vi "Write FXP.vi"(7 "FXP Configuration":T1, 8 "error in":errorcluster, 9 "DBL Value":dbl, 10 "register name":string, 11 "session in":u32) -> (0 "error out":errorcluster, 3 "session out":u32)   [LabVIEW 2018, in "FPGA Register IO.lvlib"]
uses:
  FPGA Register IO.lvlib
  TypeDefs/FXP Configuration.ctl
  <vilib>/fxp/LVFixedPointRepBitsTypeDef.ctl
  <vilib>/fxp/LVFixedPointRepRangeTypeDef.ctl
  Utilities/Find Register Offset.vi
  SubVIs/Check Register Data Store.vi
  Error Handling/Error 6001.vi
  Error Handling/Error 6000.vi
  Error Handling/Error 6002.vi
  Error Handling/Error 6006.vi
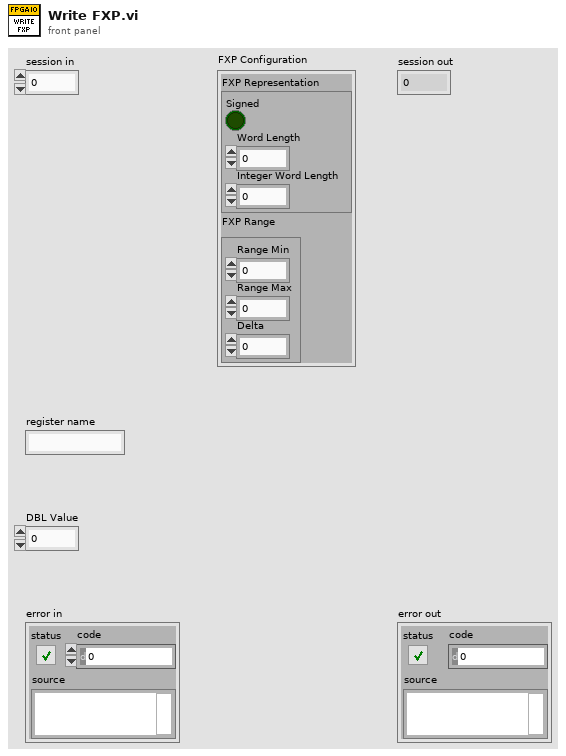
[diagram p1: front panel]
types:
  T1 = typedef "FPGA Register IO.lvlib/FXP Configuration.ctl" = cluster{"FXP Representation":T2, "FXP Range":T3}
  T2 = typedef "LVFixedPointRepBitsTypeDef.ctl" = cluster{"Signed":bool, "Word Length":u32, "Integer Word Length":i32}
  T3 = typedef "LVFixedPointRepRangeTypeDef.ctl" = cluster{"Range Min":dbl, "Range Max":dbl, "Delta":dbl}
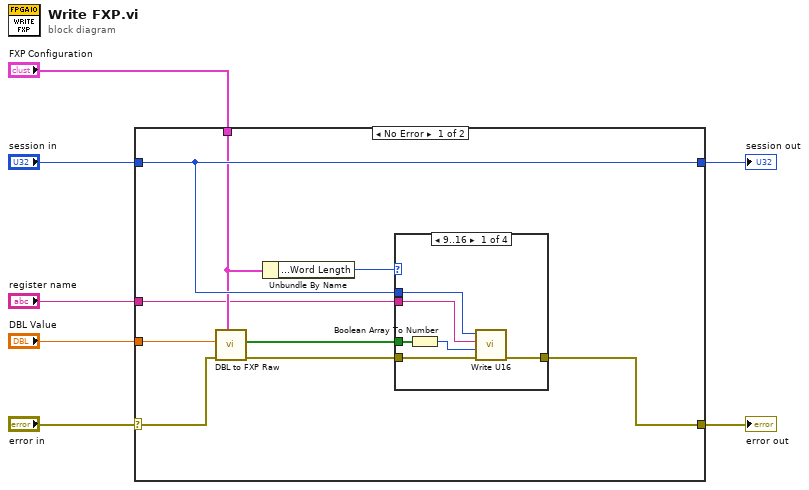
[diagram p0: block diagram]
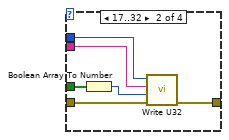
[diagram p2: hidden frame]
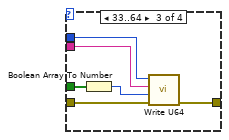
[diagram p3: hidden frame]
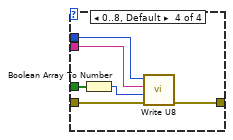
[diagram p4: hidden frame]
diagram:
  n1 = case shown="No Error" "error in" {
    selector: "error in" -> [w14 w42]
    tunnel: "session in" -> [w16 w41]
    tunnel: [w15 w42] -> w6
    tunnel: [w16 w41] -> w4
    tunnel: "FXP Configuration" -> [w9 _]
    tunnel: "DBL Value" -> [w12 _]
    tunnel: "register name" -> [w8 _]
    frame No Error {
      n2 = call "DBL to FXP Raw.vi"("FXP Configuration"=w9, "error in (no error)"=w14, "DBL Value"=w12) -> ("error out"=w13:errorcluster, "Bool Data"=w11:bool[])  [unwired: 7 in]
      n3 = Unbundle By Name(w9) -> ("FXP Representation.Word Length"=w10:u32)
      n4 = case shown="9..16" w10 {
        tunnel: w16 -> [w20 w26 w31 w39]
        tunnel: w13 -> [w22 w28 w34 w40]
        tunnel: [w21 w27 w33 w38] -> w15
        tunnel: w11 -> [w19 w25 w32 w37]
        tunnel: w8 -> [w17 w23 w29 w35]
        frame 9..16 {
          n5 = Boolean Array To Number(Boolean array=w19) -> (number=w18:u16)
          n6 = call "Write U16.vi"("error in"=w22, "value in"=w18, "register name"=w17, "session in"=w20) -> ("error out"=w21:errorcluster)  [unwired: 6 in, 1 out]
        }
        frame 17..32 {
          n7 = Boolean Array To Number(Boolean array=w25) -> (number=w24:u32)
          n8 = call "Write U32.vi"("error in"=w28, "value in"=w24, "register name"=w23, "session in"=w26) -> ("error out"=w27:errorcluster)  [unwired: 6 in, 1 out]
        }
        frame 33..64 {
          n9 = Boolean Array To Number(Boolean array=w32) -> (number=w30:u64)
          n10 = call "Write U64.vi"("error in"=w34, "value in"=w30, "register name"=w29, "session in"=w31) -> ("error out"=w33:errorcluster)  [unwired: 6 in, 1 out]
        }
        frame 0..8, Default {
          n11 = Boolean Array To Number(Boolean array=w37) -> (number=w36:u8)
          n12 = call "Write U8.vi"("error in"=w40, "value in"=w36, "register name"=w35, "session in"=w39) -> ("error out"=w38:errorcluster)  [unwired: 6 in, 1 out]
        }
      }
    }
    frame Error {
    }
  }
  "error out" <- w6
  "session out" <- w4
